vi "Initialize Bar Settings.vi"(8 "error in":errorcluster, 11 "Flex Dialog in":refnum<class "Flex UI Dialog.lvclass">) -> (0 "error out":errorcluster, 3 "Flex Dialog out":refnum<class "Flex UI Dialog.lvclass">)   [LabVIEW 2016, in "Flex UI Dialog.lvclass"]
doc: "Initializes various dialog settings."
uses:
  Flex UI Dialog.lvclass
  C:/VI Packages/Flex UI/Flex UI (Parent)/Flex UI.lvclass
  Flex UI (Parent)/Flex UI.lvclass/Flex UI.ctl
  Flex UI Dialog.lvclass/Flex UI Dialog.ctl
  Flex UI (Parent)/Flex UI.lvclass
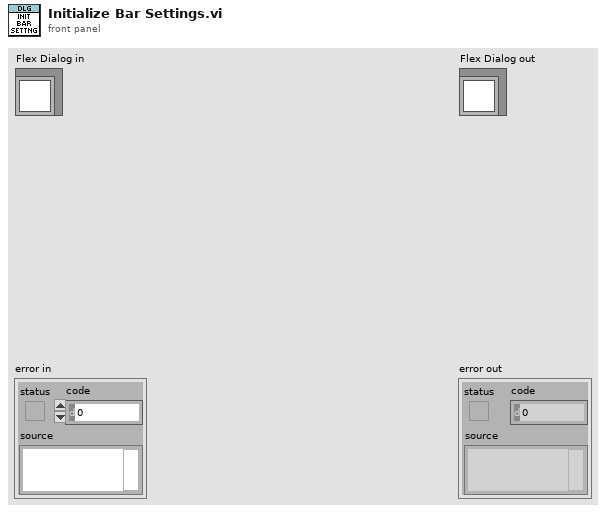
[diagram p1: front panel]
types:
  T1 = enum16{"Always On", "Always Off", "Off While Running"}
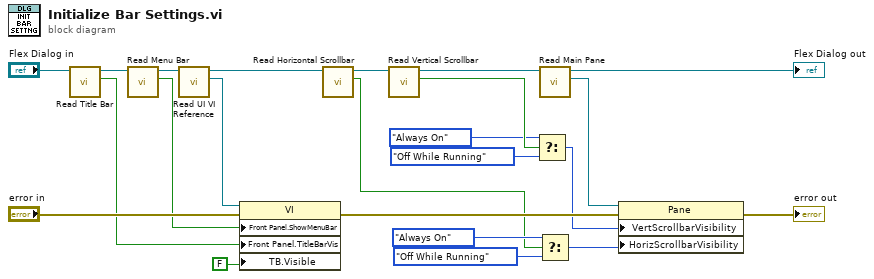
[diagram p0: block diagram]
diagram:
  n1 = call "Read Title Bar.vi"("Flex Dialog in"="Flex Dialog in") -> ("Title Bar"=w16:bool, "Flex Dialog out"=w17:refnum<class "Flex UI Dialog.lvclass">)  [unwired: 9 in]
  n2 = call "Read Menu Bar.vi"("Flex Dialog in"=w17) -> ("Menu Bar"=w18:bool, "Flex Dialog out"=w19:refnum<class "Flex UI Dialog.lvclass">)  [unwired: 9 in]
  n3 = call "Read UI VI Reference.vi"("Flex UI in"=w19) -> ("UI VI Reference"=w20:refnum<vi>, "Flex UI out"=w21:refnum<class "Flex UI Dialog.lvclass">)  [unwired: 9 in]
  n4 = property class="VI"(reference=w20, error in="error in", "Front Panel.ShowMenuBar"=w18, "Front Panel.TitleBarVis"=w16, "TB.Visible"=FALSE ("Tool Bar:Visible")) -> (error out=w11:errorcluster)  [unwired: 1 out]
  n5 = call "Read Horizontal Scrollbar.vi"("Flex Dialog in"=w21) -> ("Horizontal Scrollbar"=w1:bool, "Flex Dialog out"=w15:refnum<class "Flex UI Dialog.lvclass">)  [unwired: 9 in]
  n6 = call "Read Vertical Scrollbar.vi"("Flex Dialog in"=w15) -> ("Vertical Scrollbar"=w8:bool, "Flex Dialog out"=w14:refnum<class "Flex UI Dialog.lvclass">)  [unwired: 9 in]
  n7 = Select(t=T1."Always On" ("Vertical Scrollbar Visibility"), s=w8, f=T1."Off While Running" ("Vertical Scrollbar Visibility")) -> (s? t:f=w5:T1)
  n8 = call "Read Main Pane.vi"("Flex UI in"=w14) -> ("Main Pane"=w10:refnum<vi>, "Flex UI out"=→"Flex Dialog out":refnum<class "Flex UI Dialog.lvclass">)  [unwired: 9 in]
  n9 = Select(t=T1."Always On" ("Vertical Scrollbar Visibility"), s=w1, f=T1."Off While Running" ("Vertical Scrollbar Visibility")) -> (s? t:f=w2:T1)
  n10 = property class="Pane"(reference=w10, error in=w11, "VertScrollbarVisibility"=w5, "HorizScrollbarVisibility"=w2) -> (error out=→"error out":errorcluster)  [unwired: 1 out]
